vi "Air Heat Transfer Coefficient.vi"(4 "Cp of Air (J/kgK)":dbl, 6 "Wall Temperature (K)":dbl, 7 "Air Mass Flux (kg/s-m^2)":dbl, 9 "Air Temperature (K)":dbl, 10 "Air Re":dbl, 11 "Air Pr":dbl) -> (3 "Air Heat Xfer Coeff":dbl)   [LabVIEW 2019]
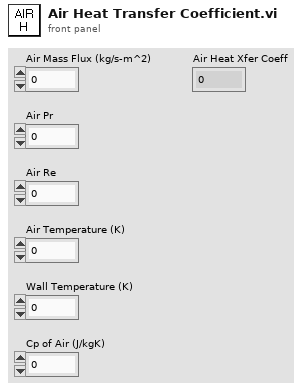
[diagram p1: front panel]
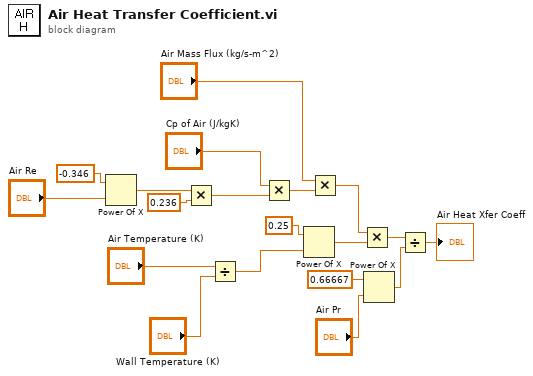
[diagram p0: block diagram]
diagram:
  n1 = Power Of X(1:"Air Re", 2:-0.346 ("y")) -> (0:w4:dbl)
  n2 = Multiply(x=w4, y=0.236) -> (x*y=w5:dbl)
  n3 = Divide(x="Air Temperature (K)", y="Wall Temperature (K)") -> (x/y=w11:dbl)
  n4 = Multiply(x="Cp of Air (J/kgK)", y=w5) -> (x*y=w7:dbl)
  n5 = Power Of X(1:w11, 2:0.25 ("y")) -> (0:w14:dbl)
  n6 = Multiply(x="Air Mass Flux (kg/s-m^2)", y=w7) -> (x*y=w13:dbl)
  n7 = Multiply(x=w13, y=w14) -> (x*y=w17:dbl)
  n8 = Power Of X(1:"Air Pr", 2:0.66667 ("y")) -> (0:w18:dbl)
  n9 = Divide(x=w17, y=w18) -> (x/y=→"Air Heat Xfer Coeff":dbl)
